vi "Sudo Wrapper.vi"(7 "Install LV Data":T1={"SSH Session"=refnum, "Status Log"="", "Detailed Log"="", "Credentials"={"Hostname or IP"="192.168.7.2", "Username"="root", "Password"=""}, "Target Info"={"OS Version"="", "CPU"="", "Systemd Version"="", "Internet Access"=FALSE, "Device Type"="", "LV Installed Ver"="", "LV Available Ver"="", "LV Upgrade Available"=FALSE, "Hostname"="", "NIC Info"=[]}, "Reboot Required?"=FALSE}, 9 "comand string":string, 11 "echo string":string) -> (3 "combined command string":string)   [LabVIEW 2019]
uses:
  <vilib>/MakerHub/LINX/Private/Utilties/Target Management/Install LV Data.ctl
  E:/lv2019/dist/vi.lib/MakerHub/LINX/Resources/Renci.SshNet.dll
  Resources/Renci.SshNet.dll
  <vilib>/MakerHub/LINX/Private/Utilties/Target Management/Target Info.ctl
  <vilib>/MakerHub/LINX/Private/Utilties/Target Management/NIC Info.ctl
  <vilib>/MakerHub/LINX/Private/Utilties/Target Management/NIC Mode.ctl
  <vilib>/MakerHub/LINX/LMH-LINX.lvlib
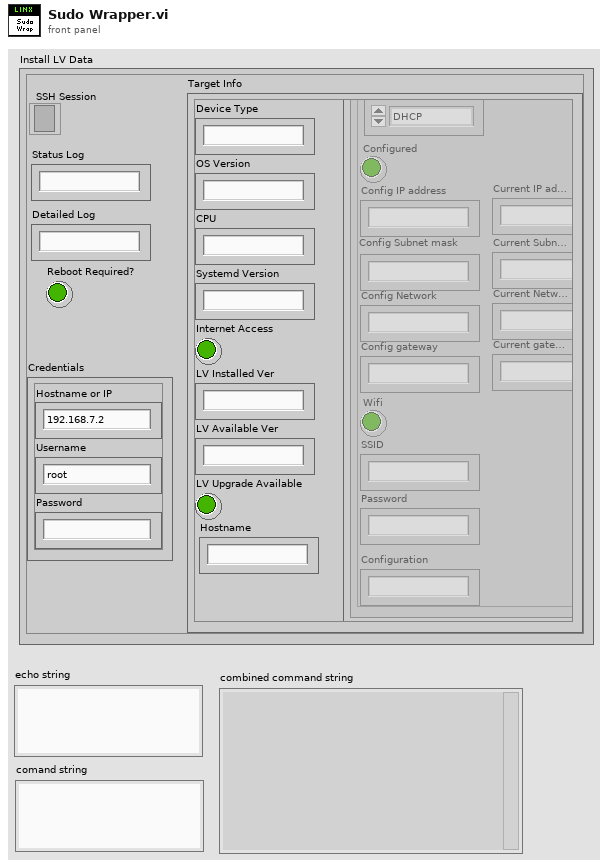
[diagram p1: front panel]
types:
  T1 = typedef "LMH-LINX.lvlib/Install LV Data.ctl" = cluster{"SSH Session":refnum<k24>, "Status Log":string, "Detailed Log":string, "Credentials":cluster{"Hostname or IP":string, "Username":string, "Password":string}, "Target Info":T2, "Reboot Required?":bool}
  T2 = typedef "LMH-LINX.lvlib/Target Info.ctl" = cluster{"OS Version":string, "CPU":string, "Systemd Version":string, "Internet Access":bool, "Device Type":string, "LV Installed Ver":string, "LV Available Ver":string, "LV Upgrade Available":bool, "Hostname":string, "NIC Info":T3[]}
  T3 = typedef "LMH-LINX.lvlib/NIC Info.ctl" = cluster{"Name":string, "NIC Mode":T4, "Configured":bool, "Config IP address":string, "Config Subnet mask":string, "Config Network":string, "Config gateway":string, "Wifi":bool, "SSID":string, "Password":string, "Configuration":string, "Current IP address":string, "Current Subnet mask":string, "Current gateway":string, "Current Network":string}
  T4 = typedef "LMH-LINX.lvlib/NIC Mode.ctl" = enum16{"DHCP", "Static", "Loopback"}
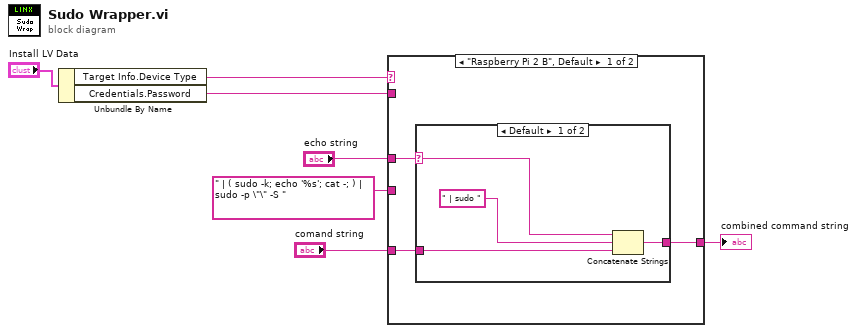
[diagram p0: block diagram]
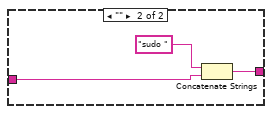
[diagram p2: hidden frame]
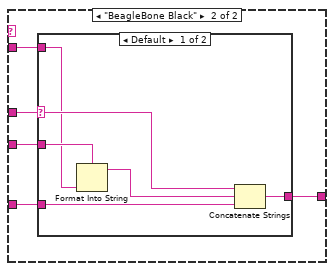
[diagram p3: hidden frame]
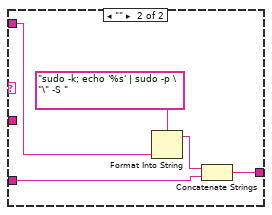
[diagram p4: hidden frame]
diagram:
  n1 = Unbundle By Name("Install LV Data") -> ("Target Info.Device Type"=w2:string, "Credentials.Password"=w1:string)
  n2 = case shown="\"Raspberry Pi 2 B\", Default" w2 {
    tunnel: "echo string" -> [w9 w22]
    tunnel: "comand string" -> [w8 w21]
    tunnel: [w10 w20] -> w5
    tunnel: " | ( sudo -k; echo '%s'; cat -; ) | sudo -p \"\" -S " ("Command") -> [_ w19]
    tunnel: w1 -> [_ w18]
    frame "Raspberry Pi 2 B", Default {
      n3 = case shown="Default" w9 {
        selector: w9 -> [w13 _]
        tunnel: w8 -> [w14 w17]
        tunnel: [w12 w16] -> w10
        frame Default {
          n4 = Concatenate Strings(w13, " | sudo " ("Command"), w14) -> (w12:string)
        }
        frame "" {
          n5 = Concatenate Strings("sudo " ("Command"), w17) -> (w16:string)
        }
      }
    }
    frame "BeagleBone Black" {
      n6 = case shown="Default" w22 {
        selector: w22 -> [w27 _]
        tunnel: w21 -> [w28 w33]
        tunnel: [w26 w32] -> w20
        tunnel: w19 -> [w25 _]
        tunnel: w18 -> [w23 w29]
        frame Default {
          n7 = Format Into String(format string=w25, w23) -> (resulting string=w24:string)  [unwired: 2 in, 1 out]
          n8 = Concatenate Strings(w27, w24, w28) -> (w26:string)
        }
        frame "" {
          n9 = Format Into String(format string="sudo -k; echo '%s' | sudo -p \"\" -S " ("Command"), w29) -> (resulting string=w31:string)  [unwired: 2 in, 1 out]
          n10 = Concatenate Strings(w31, w33) -> (w32:string)
        }
      }
    }
  }
  "combined command string" <- w5
